vi "Main.vi"() -> ()   [LabVIEW 2014]
doc: "The boiler controller allows a user to start and shut down a boiler.\n\nUse the Reset, Start, and Light Pilot controls to sequentially start the boiler. \nUse the Fuel Control Valve to change the flow of fuel into the boiler. \nUse the Stop Boiler button to shut down the boiler. \nTo shut down the system or in the event of an emergency, use the Emergency Stop button to close the application completely."
uses:
  controls/MHL Data.ctl
  controls/MHL UI Data.ctl
  controls/MHL Status.ctl
  controls/MHL References.ctl
  controls/MHL Configuration.ctl
  support/Boiler System Globals.vi
  <vilib>/Utility/error.llb/Error Cluster From Error Code.vi
  <vilib>/ErrorRing/Error Ring.xnode
  support/Message Queue/Message Queue.lvlib
  support/User Event - Stop/User Event - Stop.lvlib
  Boiler/Boiler.lvlib
panel:
  in  "Fuel Control Valve":u32(slide) min=10 max=75 scale=10.0..75.0
  in  "Stop Boiler":bool
  in  "Light Pilot":bool
  out "Forced Draft Fan":bool
  out "Pilot":bool
  out "Pilot Gas Valve":bool
  out "Primary Fan":bool
  out "Status":string
  in  "Start":bool
  in  "Reset":bool
  in  "Emergency Stop":bool
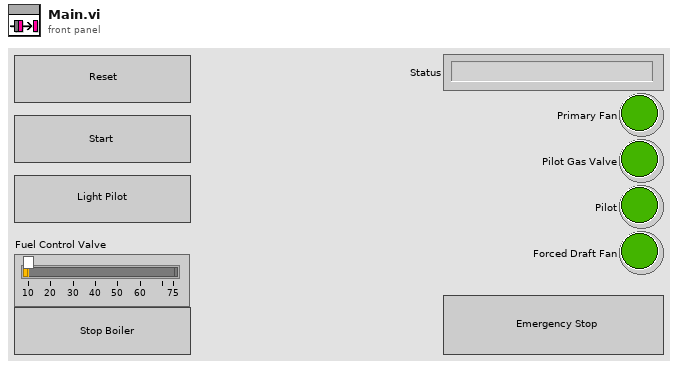
[diagram p1: front panel]
types:
  T1 = typedef "MHL Data.ctl" = cluster{"MHL User Interface Data":T2, "MHL References":T4, "MHL Configuration":T5}
  T2 = typedef "MHL UI Data.ctl" = cluster{"Status":string, "Fuel Control Valve":u32, "Primary Fan":bool, "Pilot Gas Valve":bool, "Pilot":bool, "Forced Draft Fan":bool, "MHL Status":T3}
  T3 = typedef "MHL Status.ctl" = enum16{"Lockout", "Ready", "Pre-Purge", "Pre-Purge Complete", "Pilot On", "Boiler Running", "Shutdown", "Purge"}
  T4 = typedef "MHL References.ctl" = cluster{"Reset Ref":refnum<vi>, "Start Ref":refnum<vi>, "Light Pilot Ref":refnum<vi>, "Stop Boiler Ref":refnum<vi>, "Fuel Control Valve Ref":refnum<vi>}
  T5 = typedef "MHL Configuration.ctl" = cluster{"Fuel Control Valve Maximum":dbl, "Fuel Control Valve Minimum":dbl}
  T6 = typedef "Notifiers.ctl" = cluster{"Handshake":refnum<notifier>, "Flame Level":refnum<notifier>, "Controller Exit":refnum<notifier>, "Boiler Exit":refnum<notifier>}
  T7 = typedef "Message Queue.lvlib/All Message Queues.ctl" = cluster{"MHL":refnum<queue>, "Boiler Controller":refnum<queue>, "Boiler":refnum<queue>}
  T8 = enum16{"open", "replace", "create", "open or create", "replace or create", "replace or create with confirmation"}
  T9 = enum32{"invalid app kind", "Development System", "Run Time System", "Student Edition", "Embedded LabVIEW", "Evaluation", "Custom"}
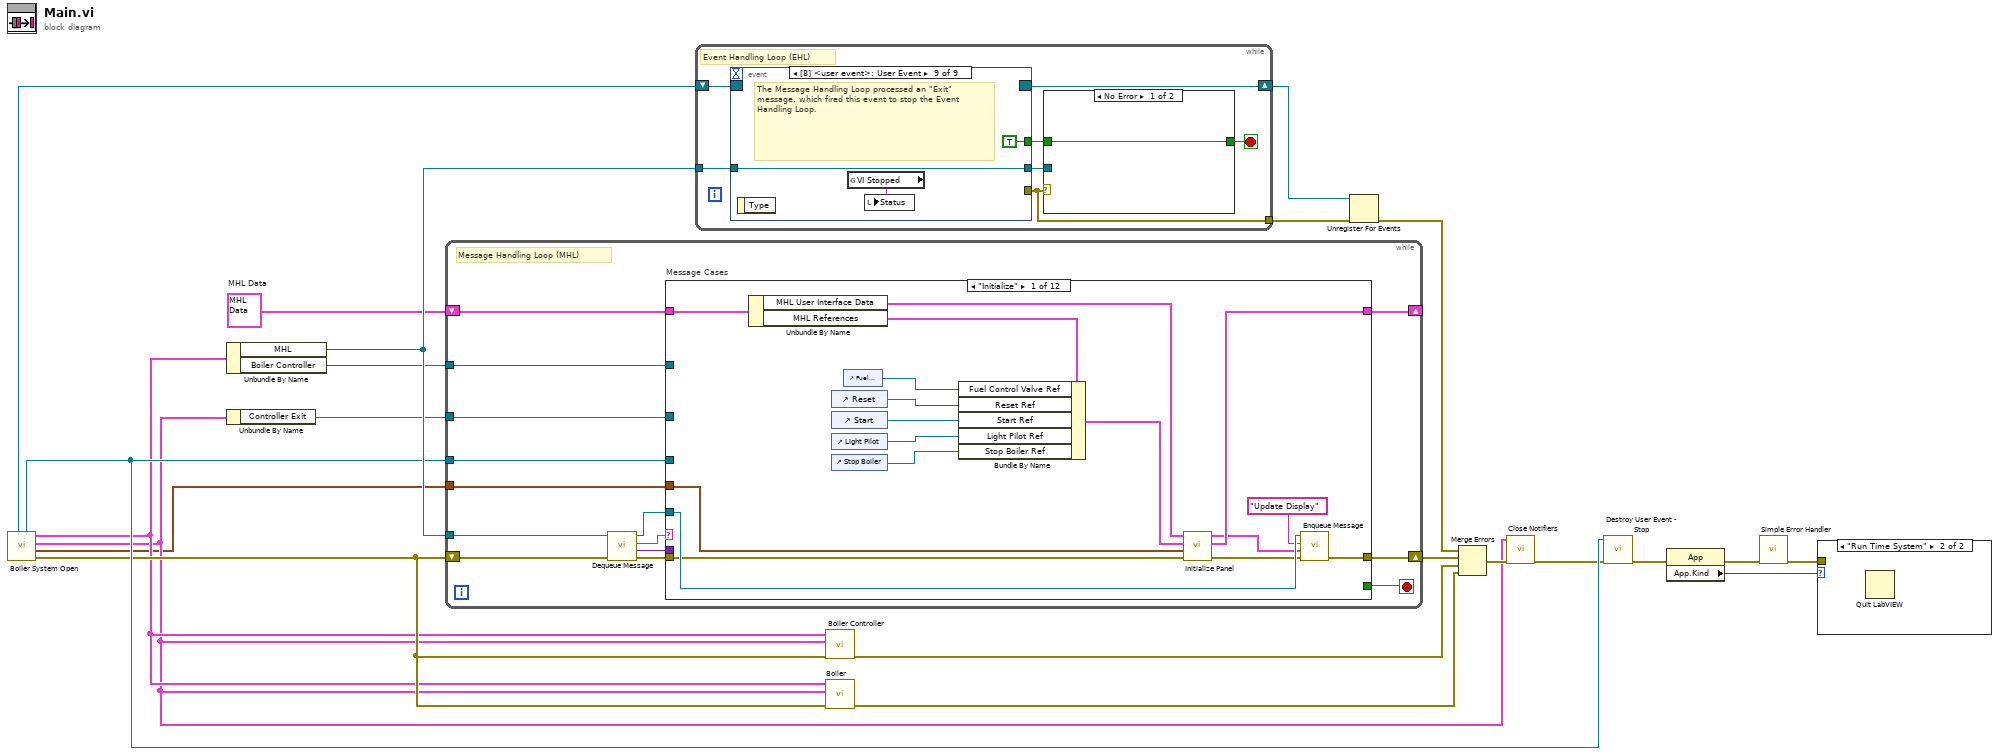
[diagram p0: block diagram]
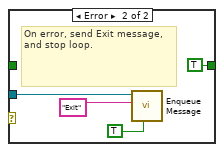
[diagram p3: hidden frame]
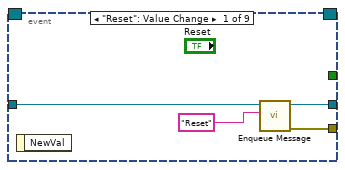
[diagram p4: hidden frame]
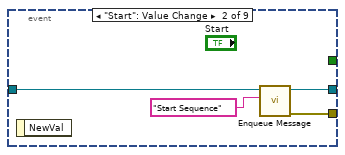
[diagram p5: hidden frame]
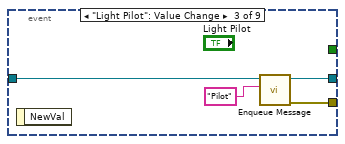
[diagram p6: hidden frame]
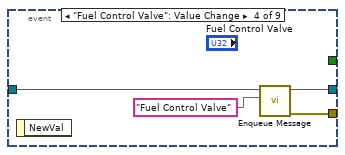
[diagram p7: hidden frame]
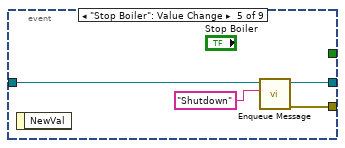
[diagram p8: hidden frame]
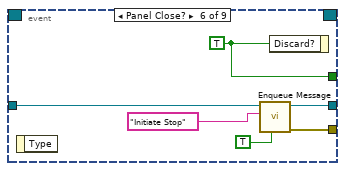
[diagram p9: hidden frame]
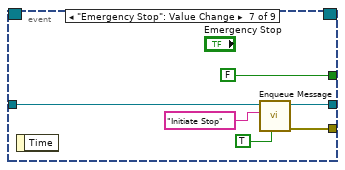
[diagram p10: hidden frame]
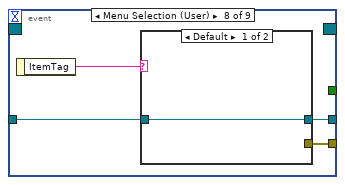
[diagram p11: hidden frame]
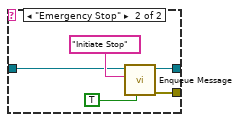
[diagram p12: hidden frame]
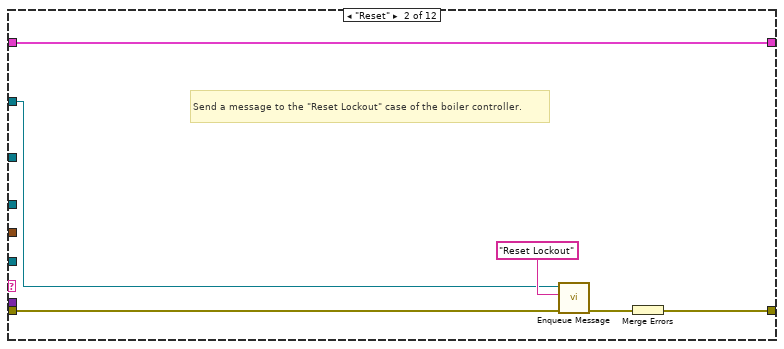
[diagram p13: hidden frame]
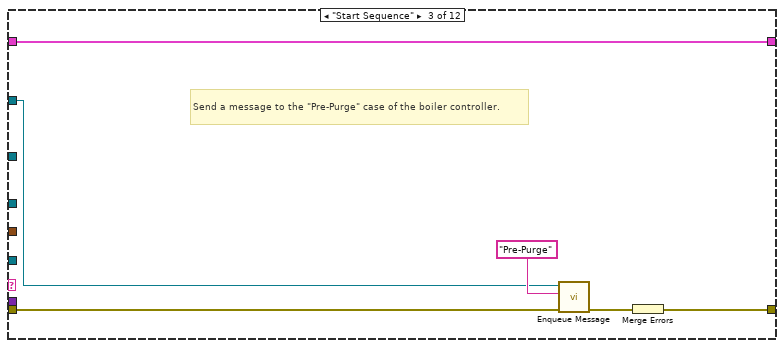
[diagram p14: hidden frame]
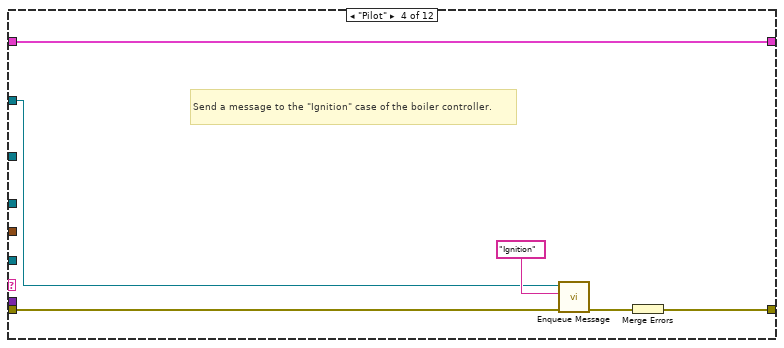
[diagram p15: hidden frame]
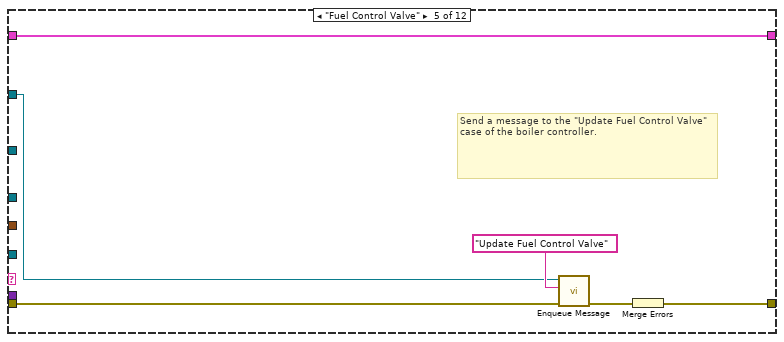
[diagram p16: hidden frame]
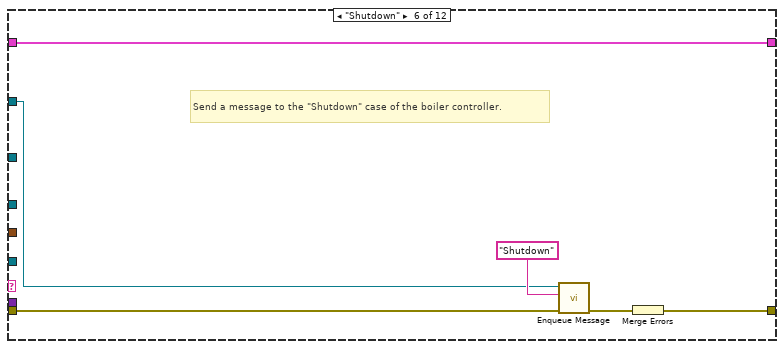
[diagram p17: hidden frame]
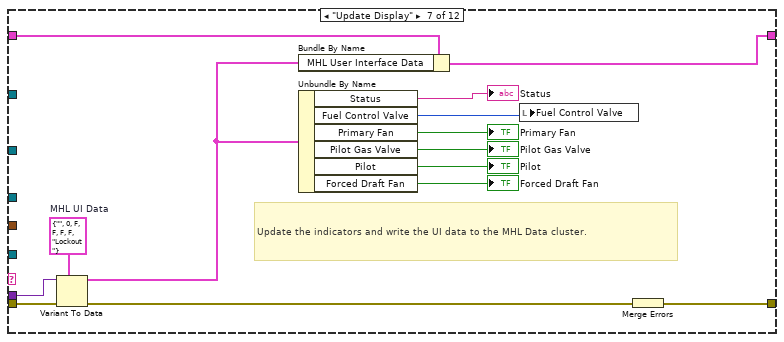
[diagram p18: hidden frame]
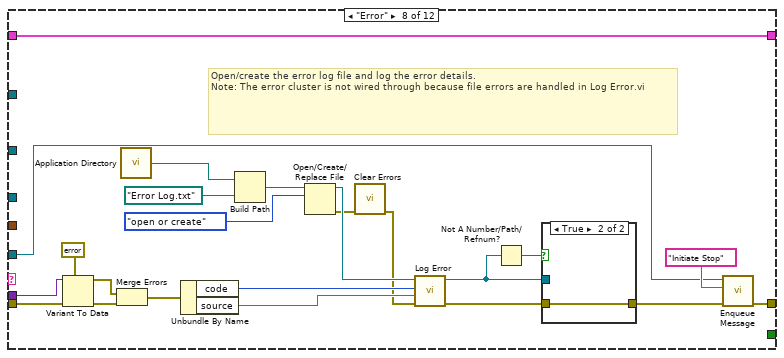
[diagram p19: hidden frame]
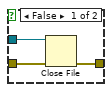
[diagram p20: hidden frame]
diagram:
  w16 = T1 {"MHL User Interface Data"={"Status"="", "Fuel Control Valve"=0, "Primary Fan"=FALSE, "Pilot Gas Valve"=FALSE, "Pilot"=FALSE, "Forced Draft Fan"=FALSE, "MHL Status"=enum."Lockout"}, "MHL References"={"Reset Ref"=refnum, "Start Ref"=refnum, "Light Pilot Ref"=refnum, "Stop Boiler Ref"=refnum, "Fuel Control Valve Ref"=refnum}, "MHL Configuration"={"Fuel Control Valve Maximum"=0.0, "Fuel Control Valve Minimum"=0.0}}  # MHL Data
  n1 = call "Boiler System Open.vi"() -> ("error out"=w7:errorcluster, "MHL Configuration"=w1:T5, "Notifiers"=w2:T6, "Message Queues"=w6:T7, "User Event - Stop"=w9:refnum<user-event>, "Stop Event Registration Refnum"=w10:refnum<event-registration>)  [unwired: 6 in]
  n2 = Unbundle By Name(w6) -> ("MHL"=w21:refnum<queue>, "Boiler Controller"=w14:refnum<queue>)
  n3 = Unbundle By Name(w2) -> ("Controller Exit"=w8:refnum<notifier>)
  n4 = while {
    tunnel: w21 -> [w26]
    shift-right: [w35] -> _
    shift-left: w16 -> [w36]
    tunnel: w9 -> [w32]
    shift-right: [w33] -> w22
    shift-left: w7 -> [w31]
    tunnel: w14 -> [w25]
    tunnel: w8 -> [w24]
    tunnel: w1 -> [w23]
    stop <- w34 stop-if-true
    # "Message Handling Loop (MHL)"
    n5 = call "Dequeue Message.vi"("error in (no error)"=w31, "Message Queue"=w26) -> ("error out"=w30:errorcluster, "Message Data"=w28:variant, "Message"=w29:string, "dup Message Queue"=w27:refnum<queue>)  [unwired: 6 in]
    n6 = case "Message Cases" shown="\"Initialize\"" w29 {
      selector: w29 -> [_ _ _ _ _ _ _ _ _ _ _ w158]
      tunnel: w27 -> [w46 _ _ _ _ _ _ w106 w127 w134 w156 _]
      tunnel: w30 -> [w40 w57 w63 w69 w72 w81 w96 w104 w132 w136 w149 _]
      tunnel: [w47 w58 w64 w70 w77 w82 w97 w102 w129 w135 w152 w157] -> w33
      tunnel: w36 -> [w48 w59 w65 w71 w73 w83 w86 w120 w131 w140 w155 w159]
      tunnel: [w38 w59 w65 w71 w73 w83 w84 w120 w131 w140 w155 w159] -> w35
      tunnel: [_ _ _ _ _ _ _ _ _ _ TRUE _] -> w34
      tunnel: w28 -> [_ _ _ _ _ _ w95 w103 _ _ _ _]
      tunnel: w32 -> [_ _ _ _ _ _ _ _ _ _ w151 _]
      tunnel: w25 -> [_ w54 w60 w66 w74 w78 _ _ w128 _ _ _]
      tunnel: w24 -> [_ _ _ _ _ _ _ _ _ w133 _ _]
      tunnel: w23 -> [w44 _ _ _ _ _ _ _ _ _ _ _]
      frame "Initialize" {
        n7 = Unbundle By Name(w48) -> ("MHL User Interface Data"=w41:T2, "MHL References"=w42:T4)
        n8 = control-ref of="Reset"() -> (w50:refnum<vi>)
        n9 = control-ref of="Start"() -> (w51:refnum<vi>)
        n10 = control-ref of="Light Pilot"() -> (w52:refnum<vi>)
        n11 = control-ref of="Stop Boiler"() -> (w53:refnum<vi>)
        n12 = control-ref of="Fuel Control Valve"() -> (w49:refnum<vi>)
        n13 = Bundle By Name(cluster=w42, "Fuel Control Valve Ref"=w49, "Reset Ref"=w50, "Start Ref"=w51, "Light Pilot Ref"=w52, "Stop Boiler Ref"=w53) -> (w43:T4)
        n14 = call "Initialize Panel.vi"("error in"=w40, "MHL Configuration"=w44, "MHL References"=w43, "MHL UI Data in"=w41) -> ("error out"=w39:errorcluster, "MHL Data out"=w38:T1, "MHL UI Data out"=w37:T2)  [unwired: 5 in]
        n15 = call "Enqueue Message.vi"("error in (no error)"=w39, "Message Data"=w37, "Message"="Update Display", "Message Queue"=w46) -> ("error out"=w47:errorcluster)  [unwired: 6 in, 1 out]
      }
      frame "Reset" {
        # "Send a message to the \"Reset Lockout\" case of the boiler controller."
        n16 = call "Enqueue Message.vi"("error in (no error)"=w57, "Message"="Reset Lockout", "Message Queue"=w54) -> ("error out"=w56:errorcluster)  [unwired: 7 in, 1 out]
        n17 = Merge Errors(w56) -> (w58:errorcluster)
      }
      frame "Start Sequence" {
        # "Send a message to the \"Pre-Purge\" case of the boiler controller."
        n18 = call "Enqueue Message.vi"("error in (no error)"=w63, "Message"="Pre-Purge", "Message Queue"=w60) -> ("error out"=w62:errorcluster)  [unwired: 7 in, 1 out]
        n19 = Merge Errors(w62) -> (w64:errorcluster)
      }
      frame "Pilot" {
        # "Send a message to the \"Ignition\" case of the boiler controller."
        n20 = call "Enqueue Message.vi"("error in (no error)"=w69, "Message"="Ignition", "Message Queue"=w66) -> ("error out"=w68:errorcluster)  [unwired: 7 in, 1 out]
        n21 = Merge Errors(w68) -> (w70:errorcluster)
      }
      frame "Fuel Control Valve" {
        # "Send a message to the \"Update Fuel Control Valve\" case of the boiler controller."
        n22 = call "Enqueue Message.vi"("error in (no error)"=w72, "Message"="Update Fuel Control Valve", "Message Queue"=w74) -> ("error out"=w76:errorcluster)  [unwired: 7 in, 1 out]
        n23 = Merge Errors(w76) -> (w77:errorcluster)
      }
      frame "Shutdown" {
        # "Send a message to the \"Shutdown\" case of the boiler controller."
        n24 = call "Enqueue Message.vi"("error in (no error)"=w81, "Message"="Shutdown", "Message Queue"=w78) -> ("error out"=w80:errorcluster)  [unwired: 7 in, 1 out]
        n25 = Merge Errors(w80) -> (w82:errorcluster)
      }
      frame "Update Display" {
        w93 = T2 {"Status"="", "Fuel Control Valve"=0, "Primary Fan"=FALSE, "Pilot Gas Valve"=FALSE, "Pilot"=FALSE, "Forced Draft Fan"=FALSE, "MHL Status"=enum."Lockout"}  # MHL UI Data
        # "Update the indicators and write the UI data to the MHL Data cluster."
        n26 = Variant To Data(error in=w96, type=w93, Variant=w95) -> (data=w85:T2, error out=w94:errorcluster)
        n27 = Bundle By Name(cluster=w86, "MHL User Interface Data"=w85) -> (w84:T1)
        n28 = Unbundle By Name(w85) -> ("Status"=→"Status":string, "Fuel Control Valve"=w91:u32, "Primary Fan"=→"Primary Fan":bool, "Pilot Gas Valve"=→"Pilot Gas Valve":bool, "Pilot"=→"Pilot":bool, "Forced Draft Fan"=→"Forced Draft Fan":bool)
        n29 = local write "Fuel Control Valve"(w91) -> ()
        n30 = Merge Errors(w94) -> (w97:errorcluster)
      }
      frame "Error" {
        # "Open/create the error log file and log the error details.\nNote: The error cluster is not wired through because file errors are handled in Log Error.vi"
        n31 = Variant To Data(error in=w104, type=errorcluster {"status"=FALSE, "code"=0, "source"=""} ("error out"), Variant=w103) -> (data=w116:errorcluster, error out=w117:errorcluster)
        n32 = Merge Errors(w116, w117) -> (w115:errorcluster)
        n33 = call <vilib>:"Application Directory.vi"() -> ("Application Directory"=w114:path)
        n34 = Unbundle By Name(w115) -> ("code"=w109:i32, "source"=w108:string)
        n35 = Build Path(base path=w114, name or relative path=path "Error Log.txt") -> (appended path=w113:path)
        n36 = Open/Create/Replace File(file path (use dialog)=w113, operation (0:open)=T8."open or create") -> (refnum out=w111:refnum<file>, error out=w99:errorcluster)  [unwired: 4 in, 1 out]
        n37 = call <vilib>:"Clear Errors.vi"("error in (no error)"=w99) -> ("error out"=w98:errorcluster)  [unwired: 5 in, 1 out]
        n38 = call "Log Error.vi"("error in"=w98, "Source"=w108, "Code"=w109, "Error Log Refnum In"=w111) -> ("error out"=w110:errorcluster, "Error Log Refnum Out"=w101:refnum<file>)  [unwired: 6 in]
        n39 = Not A Number/Path/Refnum?(number/path/refnum=w101) -> (NaN/Path/Refnum?=w100:bool)
        n40 = case shown="True" w100 {
          tunnel: w110 -> [w123 w124]
          tunnel: w101 -> [w122 _]
          tunnel: [w121 w124] -> w107
          frame False {
            n41 = Close File(refnum=w122, error in=w123) -> (error out=w121:errorcluster)  [unwired: 1 out]
          }
          frame True {
          }
        }
        n42 = call "Enqueue Message.vi"("error in (no error)"=w107, "Message"="Initiate Stop", "Message Queue"=w106) -> ("error out"=w102:errorcluster)  [unwired: 7 in, 1 out]
      }
      frame "Initiate Stop" {
        # "When stopping, first send a message to stop the boiler controller. Then wait for the boiler and boiler controller to exit."
        n43 = call "Enqueue Message.vi"("error in (no error)"=w132, "Message"="Exit", "Message Queue"=w128) -> ("error out"=w130:errorcluster)  [unwired: 7 in, 1 out]
        n44 = call "Enqueue Message.vi"("error in (no error)"=w130, "Message"="Wait on Boiler Exit", "Message Queue"=w127) -> ("error out"=w129:errorcluster)  [unwired: 7 in, 1 out]
      }
      frame "Wait on Boiler Exit" {
        # "Monitor the boiler controller to determine if it has completed its Exit. Wait 10 milliseconds for the boiler controller to respond. \nIf the notification does not occur, then enqueue another Wait on Boiler Exit message.\nIf the notification occurs, then exit the Message Handling Loop."
        n45 = Wait on Notification(notifier=w133, timeout in ms (-1)=10, error in (no error)=w136) -> (timed out?=w138:bool, error out=w137:errorcluster)  [unwired: 1 in, 2 out]
        n46 = case shown="True" w138 {
          tunnel: w137 -> [w144 w148]
          tunnel: w134 -> [w143 w146]
          tunnel: [w141 w147] -> w135
          frame False {
            n47 = call "Enqueue Message.vi"("error in (no error)"=w144, "Message"="Exit", "Message Queue"=w143) -> ("error out"=w141:errorcluster)  [unwired: 7 in, 1 out]
          }
          frame True {
            n48 = call "Enqueue Message.vi"("error in (no error)"=w148, "Message"="Wait on Boiler Exit", "Message Queue"=w146) -> ("error out"=w147:errorcluster)  [unwired: 7 in, 1 out]
          }
        }
      }
      frame "Exit" {
        # "Stop the VI"
        # "Release the message queue reference"
        n49 = call "Fire User Event - Stop.vi"("User Event - Stop"=w151) -> ("error out"=w150:errorcluster)  [unwired: 10 in]
        n50 = Release Queue(queue=w156, error in (no error)=w149) -> (error out=w153:errorcluster)  [unwired: 1 in, 2 out]
        n51 = Merge Errors(w150, w153) -> (w152:errorcluster)
      }
      frame Default {
        # "'Default' case only runs if there is a message that isn't defined in any of the other cases.  Output a programming error."
        n52 = xnode "Error Ring"("parameter 0"=w158) -> ("error out"=w157:errorcluster)
      }
    }
  }
  n53 = while {
    tunnel: w21 -> [w173]
    tunnel: [w169] -> w18
    shift-right: [w167] -> w17
    shift-left: w10 -> [w168]
    stop <- w171 stop-if-true
    # "Event Handling Loop (EHL)"
    n54 = event shown="[8] <user event>: User Event" {
      selector: w168 -> [_ _ _ _ _ _ _ _ _]
      dyn-events: [_ _ _ _ _ _ _ _ _] -> w167
      timeout: _ -> [_ _ _ _ _ _ _ _ _]
      tunnel: [_ _ _ _ _ w204 FALSE ("Discard?") _ TRUE ("Discard?")] -> w172
      tunnel: w173 -> [w182 w186 w190 w194 w198 w203 w210 w213 w223]
      tunnel: [w181 w184 w188 w192 w196 w202 w209 w211 _] -> w169
      tunnel: [w180 w185 w189 w193 w197 w201 w207 w212 w223] -> w170
      event "Reset": Value Change {
        n55 = event-data() -> ()  [unwired: 1 in, 1 out]
        n56 = call "Enqueue Message.vi"("Message"="Reset", "Message Queue"=w182) -> ("error out"=w181:errorcluster, "dup Message Queue"=w180:refnum<queue>)  [unwired: 8 in]
      }
      event "Start": Value Change {
        n57 = event-data() -> ()  [unwired: 1 in, 1 out]
        n58 = call "Enqueue Message.vi"("Message"="Start Sequence", "Message Queue"=w186) -> ("error out"=w184:errorcluster, "dup Message Queue"=w185:refnum<queue>)  [unwired: 8 in]
      }
      event "Light Pilot": Value Change {
        n59 = event-data() -> ()  [unwired: 1 in, 1 out]
        n60 = call "Enqueue Message.vi"("Message"="Pilot", "Message Queue"=w190) -> ("error out"=w188:errorcluster, "dup Message Queue"=w189:refnum<queue>)  [unwired: 8 in]
      }
      event "Fuel Control Valve": Value Change {
        n61 = event-data() -> ()  [unwired: 1 in, 1 out]
        n62 = call "Enqueue Message.vi"("Message"="Fuel Control Valve", "Message Queue"=w194) -> ("error out"=w192:errorcluster, "dup Message Queue"=w193:refnum<queue>)  [unwired: 8 in]
      }
      event "Stop Boiler": Value Change {
        n63 = event-data() -> ()  [unwired: 1 in, 1 out]
        n64 = call "Enqueue Message.vi"("Message"="Shutdown", "Message Queue"=w198) -> ("error out"=w196:errorcluster, "dup Message Queue"=w197:refnum<queue>)  [unwired: 8 in]
      }
      event Panel Close? {
        w204 = TRUE ("Discard?")
        n65 = event-data() -> ()  [unwired: 1 in, 1 out]
        n66 = call "Enqueue Message.vi"("Priority Message? (F)"=TRUE, "Message"="Initiate Stop", "Message Queue"=w203) -> ("error out"=w202:errorcluster, "dup Message Queue"=w201:refnum<queue>)  [unwired: 7 in]
        n67 = event-data("Discard?"=w204) -> ()  [unwired: 1 in, 1 out]
      }
      event "Emergency Stop": Value Change {
        n68 = event-data() -> ()  [unwired: 1 in, 1 out]
        n69 = call "Enqueue Message.vi"("Priority Message? (F)"=TRUE, "Message"="Initiate Stop", "Message Queue"=w210) -> ("error out"=w209:errorcluster, "dup Message Queue"=w207:refnum<queue>)  [unwired: 7 in]
      }
      event Menu Selection (User) {
        n70 = event-data() -> ("ItemTag"=w214:string)  [unwired: 1 in]
        n71 = case shown="Default" w214 {
          tunnel: w213 -> [w215 w218]
          tunnel: [w215 w217] -> w212
          tunnel: [_ w216] -> w211
          frame Default {
          }
          frame "Emergency Stop" {
            n72 = call "Enqueue Message.vi"("Priority Message? (F)"=TRUE, "Message"="Initiate Stop", "Message Queue"=w218) -> ("error out"=w216:errorcluster, "dup Message Queue"=w217:refnum<queue>)  [unwired: 7 in]
          }
        }
      }
      event User Event {
        # "The Message Handling Loop processed an \"Exit\" message, which fired this event to stop the Event Handling Loop."
        n73 = event-data() -> ()  [unwired: 1 in, 1 out]
        n74 = global read "Boiler System Globals.vi" "VI Stopped"() -> (w221:string)
        n75 = local write "Status"(w221) -> ()
      }
    }
    n76 = case shown="No Error" w169 {
      tunnel: [w174 TRUE ("Discard?")] -> w171
      tunnel: w172 -> [w174 _]
      tunnel: w170 -> [_ w177]
      frame No Error {
      }
      frame Error {
        # "On error, send Exit message, and stop loop."
        n77 = call "Enqueue Message.vi"("Priority Message? (F)"=TRUE, "Message"="Exit", "Message Queue"=w177) -> ()  [unwired: 7 in, 2 out]
      }
    }
  }
  n78 = call "Boiler Controller.vi"("error in"=w7, "Notifiers"=w2, "Message Queues"=w6) -> ("error out"=w15:errorcluster)  [unwired: 8 in]
  n79 = call "Boiler.vi"("error in"=w7, "Notifiers"=w2, "Message Queues"=w6) -> ("error out"=w5:errorcluster)  [unwired: 8 in]
  n80 = Unregister For Events(event registration refnum=w17, error in=w18) -> (error out=w19:errorcluster)
  n81 = Merge Errors(w19, w22, w15, w5) -> (w4:errorcluster)
  n82 = call "Close Notifiers.vi"("error in"=w4, "Notifiers"=w2) -> ("error out"=w3:errorcluster)  [unwired: 9 in]
  n83 = call "Destroy User Event - Stop.vi"("error in (no error)"=w3, "User Event - Stop"=w9) -> ("error out"=w20:errorcluster)  [unwired: 9 in]
  n84 = property class="App"(error in=w20) -> (error out=w13:errorcluster, "App.Kind"=w12:T9)  [unwired: 1 in, 1 out]
  n85 = call <vilib>:"Simple Error Handler.vi"("error in (no error)"=w13) -> ("error out"=w11:errorcluster)  [unwired: 4 in, 4 out]
  n86 = case shown="\"Run Time System\"" w12 {
    tunnel: w11 -> [_ _]
    frame Default {
    }
    frame "Run Time System" {
      n87 = Quit LabVIEW() -> ()  [unwired: 1 in]
    }
  }
